vi "Dialog Box.vi"(8 "error in (no error)":errorcluster, 11 "MessageBox in":refnum<class "MessageBox.lvclass">) -> (0 "error out":errorcluster, 1 "timed out?":bool, 2 "Selection":string, 3 "MessageBox out":refnum<class "MessageBox.lvclass">)   [LabVIEW 2012, in "MessageBox.lvlib" / "MessageBox.lvclass"]
doc: "This VI contains the code for the dialog box.\nOverride this VI to provide more functionality or to create your own application-specific dialog box."
uses:
  MessageBox.lvclass
  <vilib>/Utility/miscctls.llb/LVBoundsTypeDef.ctl
  <vilib>/Utility/miscctls.llb/LVPositionTypeDef.ctl
  Fading/_Fade In(I32).vi
panel:
  out "Picture":picture
  out "String":string
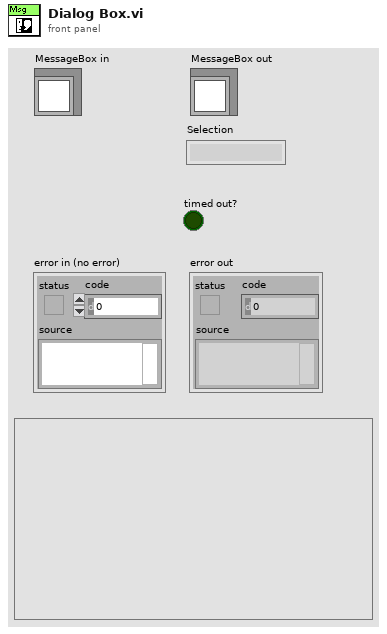
[diagram p1: front panel]
types:
  T1 = typedef "LVPositionTypeDef.ctl" = cluster{"Left":i32, "Top":i32}
  T2 = typedef "LVBoundsTypeDef.ctl" = cluster{"Width":u32, "Height":u32}
  T3 = typedef "imagedata.ctl" = cluster{"image type":i32, "image depth":i32, "image":u8[], "mask":u8[], "colors":u32[], "Rectangle":cluster{"left":i16, "top":i16, "right":i16, "bottom":i16}}
  T4 = cluster{"left":i16, "top":i16, "right":i16, "bottom":i16}
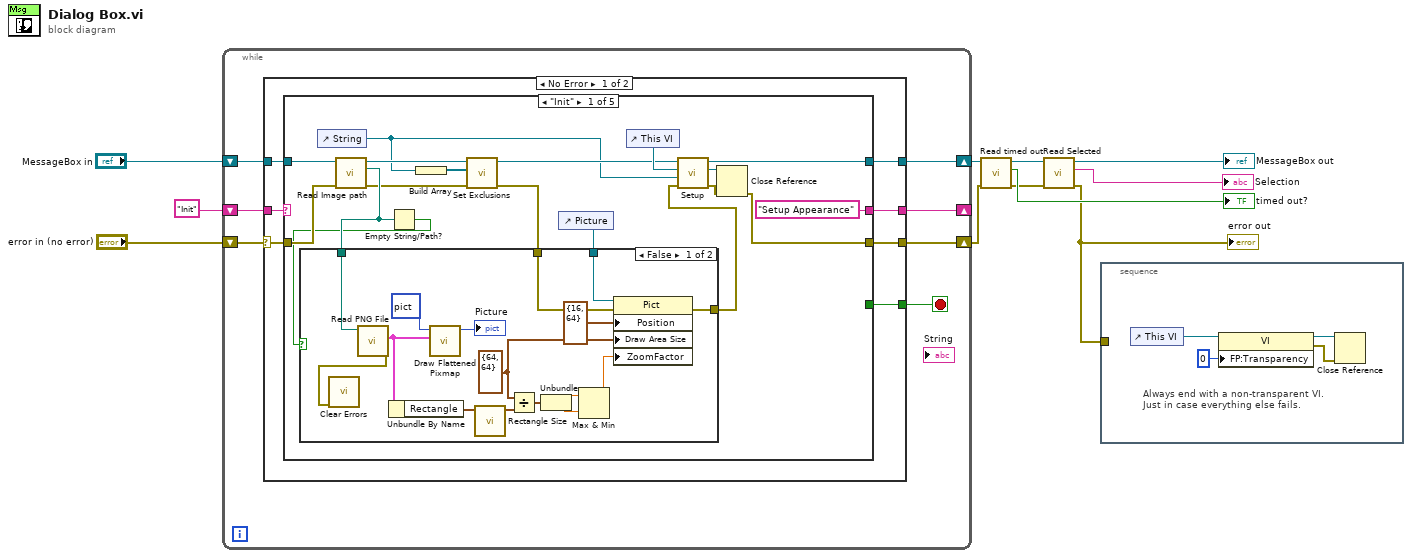
[diagram p0: block diagram]
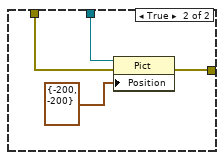
[diagram p2: hidden frame]
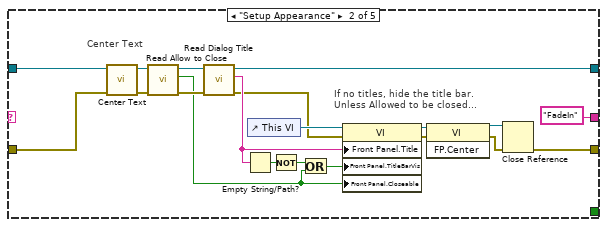
[diagram p3: hidden frame]
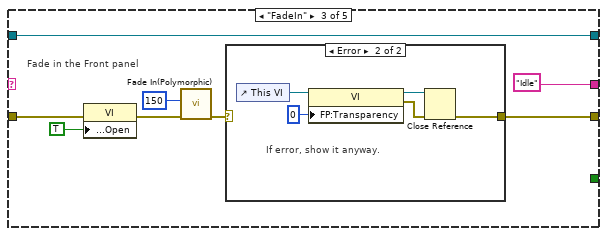
[diagram p4: hidden frame]
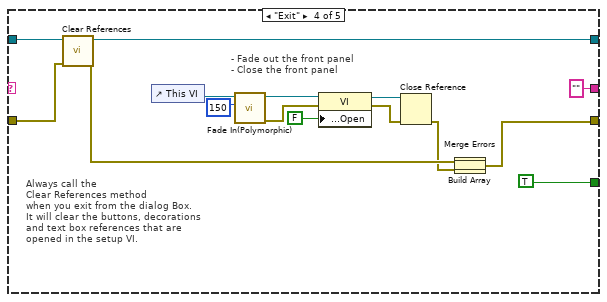
[diagram p6: hidden frame]
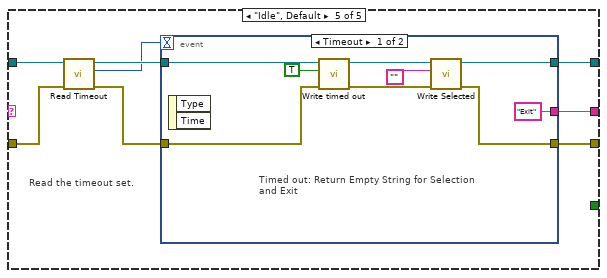
[diagram p7: hidden frame]
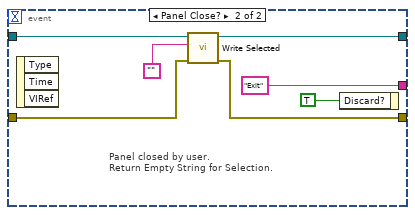
[diagram p8: hidden frame]
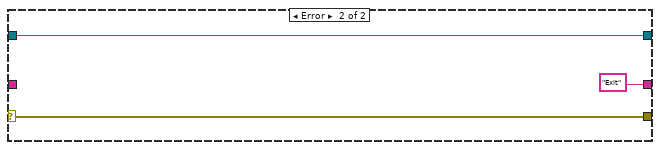
[diagram p9: hidden frame]
diagram:
  n1 = while {
    shift-right: [w14] -> _
    shift-left: "Init" -> [w15]
    shift-right: [w18] -> w4
    shift-left: "MessageBox in" -> [w17]
    shift-right: [w16] -> w3
    shift-left: "error in (no error)" -> [w12]
    stop <- w13 stop-if-true
    n2 = case shown="No Error" w12 {
      selector: w12 -> [w19 w138]
      tunnel: [w25 w140] -> w18
      tunnel: w17 -> [w24 w140]
      tunnel: [w23 w138] -> w16
      tunnel: w15 -> [w22 _]
      tunnel: [w21 "Exit"] -> w14
      tunnel: [w20 _] -> w13
      frame No Error {
        n3 = case shown="\"Init\"" w22 {
          tunnel: [w41 w74 w91 w103 w121] -> w25
          tunnel: w24 -> [w31 w72 w91 w104 w118]
          tunnel: [w38 w75 w87 w99 w120] -> w23
          tunnel: w19 -> [w37 w71 w86 w102 w115]
          tunnel: ["Setup Appearance" "FadeIn" "Idle" "" w119] -> w21
          tunnel: [_ _ _ TRUE _] -> w20
          frame "Init" {
            n4 = control-ref of="String"() -> (w26:refnum<vi>)
            n5 = call-dynamic "Read Image path.vi"("error in (no error)"=w37, "MessageBox.lvclass in"=w31) -> ("error out"=w28:errorcluster, "Image path"=w36:path, "MessageBox.lvclass out"=w32:refnum<class "MessageBox.lvclass">)  [unwired: 7 out]
            n6 = Empty String/Path?(string/path=w36) -> (empty?=w34:bool)
            n7 = Build Array(w26) -> (w27:refnum<vi>[])
            n8 = call-dynamic "Set Exclusions.vi"("error in (no error)"=w28, "Exclusions"=w27, "Dialog in"=w32) -> ("error out"=w29:errorcluster, "Dialog out"=w30:refnum<class "MessageBox.lvclass">)  [unwired: 7 out]
            n9 = control-ref of="Picture"() -> (w33:refnum<vi>)
            n10 = case shown="False" w34 {
              tunnel: w36 -> [w49 _]
              tunnel: [w47 w63] -> w35
              tunnel: w29 -> [w46 w62]
              tunnel: w33 -> [w44 w61]
              frame False {
                w59 = T2 {"Width"=64, "Height"=64} ("Draw Area Size")
                n11 = call <vilib>:"Read PNG File.vi"("path to PNG file"=w49) -> ("error out"=w48:errorcluster, "image data"=w52:T3)  [unwired: 1 in, 8 out]
                n12 = call <vilib>:"Clear Errors.vi"("error in (no error)"=w48) -> ()  [unwired: 7 out]
                n13 = Unbundle By Name(w52) -> ("Rectangle"=w53:T4)
                n14 = call <vilib>:"Draw Flattened Pixmap.vi"("image data"=w52, "picture"=picture data[5B]) -> ("new picture"=→"Picture":picture)  [unwired: 7 out]
                n15 = call "Rectangle Size.vi"("Rectangle"=w53) -> ("Rect Size"=w58:cluster{"width":i32, "height":i32})  [unwired: 10 out]
                n16 = Divide(x=w59, y=w58) -> (x/y=w54:cluster{dbl, dbl})
                n17 = Unbundle(w54) -> (w55:dbl, w56:dbl)
                n18 = Max & Min(x=w55, y=w56) -> (max(x,y)=w57:dbl)  [unwired: 1 out]
                n19 = property class="Pict"(reference=w44, error in=w46, "Position"=T1 {"Left"=16, "Top"=64}, "Draw Area Size"=w59, "ZoomFactor"=w57) -> (error out=w47:errorcluster)  [unwired: 1 out]
              }
              frame True {
                n20 = property class="Pict"(reference=w61, error in=w62, "Position"=T1 {"Left"=-200, "Top"=-200}) -> (error out=w63:errorcluster)  [unwired: 1 out]
              }
            }
            n21 = control-ref of="This VI"() -> (w42:refnum<vi>)
            n22 = call-dynamic "Setup.vi"("error in (no error)"=w35, "Str Refnum"=w26, "VI Reference"=w42, "Dialog in"=w30) -> ("error out"=w39:errorcluster, "VI reference (dup)"=w40:refnum<vi>, "Dialog out"=w41:refnum<class "MessageBox.lvclass">)  [unwired: 5 out]
            n23 = Close Reference(reference=w40, error in (no error)=w39) -> (error out=w38:errorcluster)
          }
          frame "Setup Appearance" {
            # "Center Text"
            # "If no titles, hide the title bar.\nUnless Allowed to be closed..."
            n24 = call-dynamic "Center Text.vi"("error in (no error)"=w71, "Dialog in"=w72) -> ("error out"=w68:errorcluster, "Dialog out"=w70:refnum<class "MessageBox.lvclass">)  [unwired: 8 out]
            n25 = call-dynamic "Read Allow to Close.vi"("error in (no error)"=w68, "Dialog.lvclass in"=w70) -> ("error out"=w67:errorcluster, "Allow to close?"=w64:bool, "Dialog.lvclass out"=w69:refnum<class "MessageBox.lvclass">)  [unwired: 7 out]
            n26 = call-dynamic "Read Dialog Title.vi"("error in (no error)"=w67, "Dialog in"=w69) -> ("error out"=w73:errorcluster, "Dialog Title"=w78:string, "Dialog out"=w74:refnum<class "MessageBox.lvclass">)  [unwired: 7 out]
            n27 = Empty String/Path?(string/path=w78) -> (empty?=w81:bool)
            n28 = control-ref of="This VI"() -> (w82:refnum<vi>)
            n29 = Not(x=w81) -> (.not. x?=w66:bool)
            n30 = Or(x=w66, y=w64) -> (x .or. y?=w65:bool)
            n31 = property class="VI"(reference=w82, error in=w73, "Front Panel.Title"=w78, "Front Panel.TitleBarVis"=w65, "Front Panel.Closeable"=w64) -> (reference out=w80:refnum<vi>, error out=w79:errorcluster)
            n32 = invoke class="VI" method="FP.Center"(reference=w80, error in=w79) -> (reference out=w77:refnum<vi>, error out=w76:errorcluster)  [unwired: 1 in, 1 out]
            n33 = Close Reference(reference=w77, error in (no error)=w76) -> (error out=w75:errorcluster)
          }
          frame "FadeIn" {
            # "Fade in the Front panel"
            n34 = property class="VI"(error in=w86, "Front Panel.Open"=TRUE ("Front Panel Window:Open")) -> (error out=w85:errorcluster)  [unwired: 1 in, 1 out]
            n35 = call-poly "Fade In(Polymorphic).vi"("error in"=w85, "Fade time (ms)"=150) -> ("error out"=w88:errorcluster)  [unwired: 2 in, 7 out]
            n36 = case shown="Error" w88 {
              selector: w88 -> [w92 _]
              tunnel: [w92 w93] -> w87
              frame No Error {
              }
              frame Error {
                # "If error, show it anyway."
                n37 = control-ref of="This VI"() -> (w95:refnum<vi>)
                n38 = property class="VI"(reference=w95, "FP:Transparency"=u8 0 ("Front Panel Window:Transparency")) -> (reference out=w96:refnum<vi>, error out=w97:errorcluster)  [unwired: 1 in]
                n39 = Close Reference(reference=w96, error in (no error)=w97) -> (error out=w93:errorcluster)
              }
            }
          }
          frame "Exit" {
            # "Always call the\nClear References method\nwhen you exit from the dialog Box.\nIt will clear the buttons, decorations\nand text box references that are \nopened in the setup VI."
            # "- Fade out the front panel\n- Close the front panel"
            n40 = call-dynamic "Clear References.vi"("error in (no error)"=w102, "Dialog in"=w104) -> ("error out"=w101:errorcluster, "Dialog out"=w103:refnum<class "MessageBox.lvclass">)  [unwired: 8 out]
            n41 = control-ref of="This VI"() -> (w110:refnum<vi>)
            n42 = call-poly "Fade In(Polymorphic).vi"("Fade time (ms)"=150, "VI Reference (calling VI)"=w110) -> ("error out"=w108:errorcluster, "dup VI Reference"=w109:refnum<vi>)  [unwired: 2 in, 6 out]
            n43 = property class="VI"(reference=w109, error in=w108, "Front Panel.Open"=FALSE ("Front Panel Window:Open")) -> (reference out=w106:refnum<vi>, error out=w105:errorcluster)
            n44 = Close Reference(reference=w106, error in (no error)=w105) -> (error out=w100:errorcluster)
            n45 = Build Array(w101, w100) -> (w98:errorcluster[])
            n46 = Merge Errors(w98) -> (w99:errorcluster)
          }
          frame "Idle", Default {
            # "Read the timeout set."
            n47 = call-dynamic "Read Timeout.vi"("error in (no error)"=w115, "Dialog.lvclass in"=w118) -> ("error out"=w114:errorcluster, "Timeout"=w116:i32, "Dialog.lvclass out"=w117:refnum<class "MessageBox.lvclass">)  [unwired: 7 out]
            n48 = event shown="[0] Timeout" {
              selector: _ -> [_ _]
              dyn-events: _ -> [_ _]
              timeout: w116 -> [_ _]
              tunnel: [w123 w133] -> w121
              tunnel: w117 -> [w129 w134]
              tunnel: [w124 w131] -> w120
              tunnel: w114 -> [w127 w132]
              tunnel: ["Exit" "Exit"] -> w119
              event Timeout {
                # "Timed out: Return Empty String for Selection\nand Exit"
                n49 = event-data() -> ()  [unwired: 3 out]
                n50 = call-dynamic "Write timed out.vi"("error in (no error)"=w127, "timed out?"=TRUE, "Dialog.lvclass in"=w129) -> ("error out"=w125:errorcluster, "Dialog.lvclass out"=w126:refnum<class "MessageBox.lvclass">)  [unwired: 7 out]
                n51 = call-dynamic "Write Selected.vi"("error in (no error)"=w125, "Selected"="", "Dialog.lvclass in"=w126) -> ("error out"=w124:errorcluster, "Dialog.lvclass out"=w123:refnum<class "MessageBox.lvclass">)  [unwired: 7 out]
              }
              event Panel Close? {
                # "Panel closed by user.\nReturn Empty String for Selection."
                n52 = event-data() -> ()  [unwired: 4 out]
                n53 = call-dynamic "Write Selected.vi"("error in (no error)"=w132, "Selected"="", "Dialog.lvclass in"=w134) -> ("error out"=w131:errorcluster, "Dialog.lvclass out"=w133:refnum<class "MessageBox.lvclass">)  [unwired: 7 out]
                n54 = event-data("Discard?"=TRUE) -> ()  [unwired: 1 in, 1 out]
              }
            }
          }
        }
      }
      frame Error {
      }
    }
  }
  n55 = call-dynamic "Read timed out.vi"("error in (no error)"=w3, "Dialog.lvclass in"=w4) -> ("error out"=w1:errorcluster, "timed out?"=→"timed out?":bool, "Dialog.lvclass out"=w2:refnum<class "MessageBox.lvclass">)  [unwired: 7 out]
  n56 = call-dynamic "Read Selected.vi"("error in (no error)"=w1, "Dialog.lvclass in"=w2) -> ("error out"=w6:errorcluster, "Selected"=→"Selection":string, "Dialog.lvclass out"=→"MessageBox out":refnum<class "MessageBox.lvclass">)  [unwired: 7 out]
  "error out" <- w6
  n57 = stacked-sequence {
    tunnel: w6 -> [_]
    frame #0 {
      # "Always end with a non-transparent VI.\nJust in case everything else fails."
      n58 = control-ref of="This VI"() -> (w143:refnum<vi>)
      n59 = property class="VI"(reference=w143, "FP:Transparency"=u8 0 ("Front Panel Window:Transparency")) -> (reference out=w142:refnum<vi>, error out=w141:errorcluster)  [unwired: 1 in]
      n60 = Close Reference(reference=w142, error in (no error)=w141) -> ()  [unwired: 1 out]
    }
  }
